vi "correlation calculation for trap 3 absolute positioning.vi"(3 "Number of sets to average":dbl, 4 "Accumulated array":dbl[][](array[numeric]), 5 "raw data":dbl[][](array[numeric])) -> (0 "Accumulated array out":dbl[][](array[numeric]), 1 "Y correlation":dbl, 2 "X correlation":dbl)   [LabVIEW 2014]
uses:
  <vilib>/Analysis/baseanly.llb/Mean (DBL).vi
  <vilib>/Analysis/NI_AALBase.lvlib
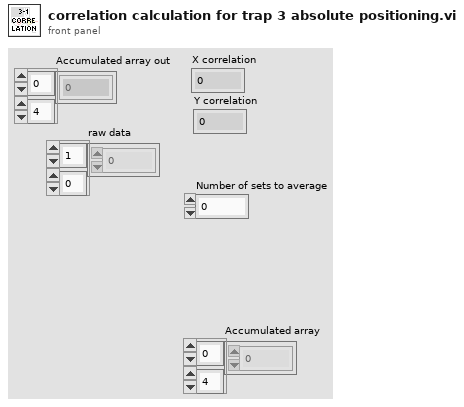
[diagram p1: front panel]
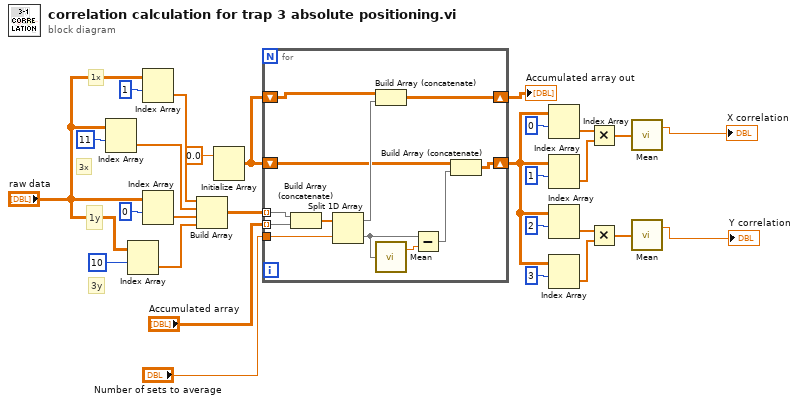
[diagram p0: block diagram]
diagram:
  # "3y"
  # "1y"
  # "3x"
  # "1x"
  n1 = Index Array(array="raw data", index (row)=11) -> (element=w22:dbl[])  [unwired: 1 in]
  n2 = Index Array(array="raw data", index (row)=10) -> (element=w20:dbl[])  [unwired: 1 in]
  n3 = Index Array(array="raw data", index (row)=1) -> (element=w23:dbl[])  [unwired: 1 in]
  n4 = Index Array(array="raw data", index (row)=0) -> (element=w21:dbl[])  [unwired: 1 in]
  n5 = Build Array(w23, w22, w21, w20) -> (w19:dbl[][])
  n6 = Initialize Array(0.0) -> (w15:dbl[][])  [unwired: 2 in]
  n7 = for {
    tunnel: w19 -> [w38] mode=indexing
    tunnel: "Accumulated array" -> [w37] mode=indexing
    tunnel: "Number of sets to average" -> [w36]
    shift-right: [w34] -> w3
    shift-left: w15 -> [w35]
    shift-right: [w29] -> w14
    shift-left: w15 -> [w31]
    n8 = Build Array (concatenate)(w38, w37) -> (w39:dbl[])
    n9 = Split 1D Array(array=w39, index=w36) -> (first subarray=w40:dbl[], second subarray=w33:dbl[])
    n10 = Build Array (concatenate)(w35, w40) -> (w34:dbl[][])
    n11 = call-poly <vilib>:"Mean.vi"("X"=w33) -> ("mean"=w32:dbl)  [unwired: 1 out]
    n12 = Subtract(x=w33, y=w32) -> (x-y=w30:dbl[])
    n13 = Build Array (concatenate)(w31, w30) -> (w29:dbl[][])
  }
  "Accumulated array out" <- w3
  n14 = Index Array(array=w14, index (row)=0) -> (element=w9:dbl[])  [unwired: 1 in]
  n15 = Index Array(array=w14, index (row)=1) -> (element=w8:dbl[])  [unwired: 1 in]
  n16 = Index Array(array=w14, index (row)=2) -> (element=w7:dbl[])  [unwired: 1 in]
  n17 = Index Array(array=w14, index (row)=3) -> (element=w6:dbl[])  [unwired: 1 in]
  n18 = Multiply(x=w9, y=w8) -> (x*y=w5:dbl[])
  n19 = Multiply(x=w7, y=w6) -> (x*y=w4:dbl[])
  n20 = call-poly <vilib>:"Mean.vi"("X"=w5) -> ("mean"=→"X correlation":dbl)  [unwired: 1 out]
  n21 = call-poly <vilib>:"Mean.vi"("X"=w4) -> ("mean"=→"Y correlation":dbl)  [unwired: 1 out]
